vi "Relay_CYL.vi"(6 "DUT":u8, 7 "EOL/FCT":bool, 8 "error out":errorcluster, 9 "DOs":bool[](array[boolean]), 10 "Relay_Channel_Out":T1[](array[typedef]), 11 "Relay":refnum<queue>) -> (0 "error out 2":errorcluster)   [LabVIEW 2024, in "Test_2.lvlib"]
uses:
  Test_2.lvlib
  Relay_Module/support/Relay_Enum_OUT.ctl
  Relay_Module/Relay_Module.lvlib
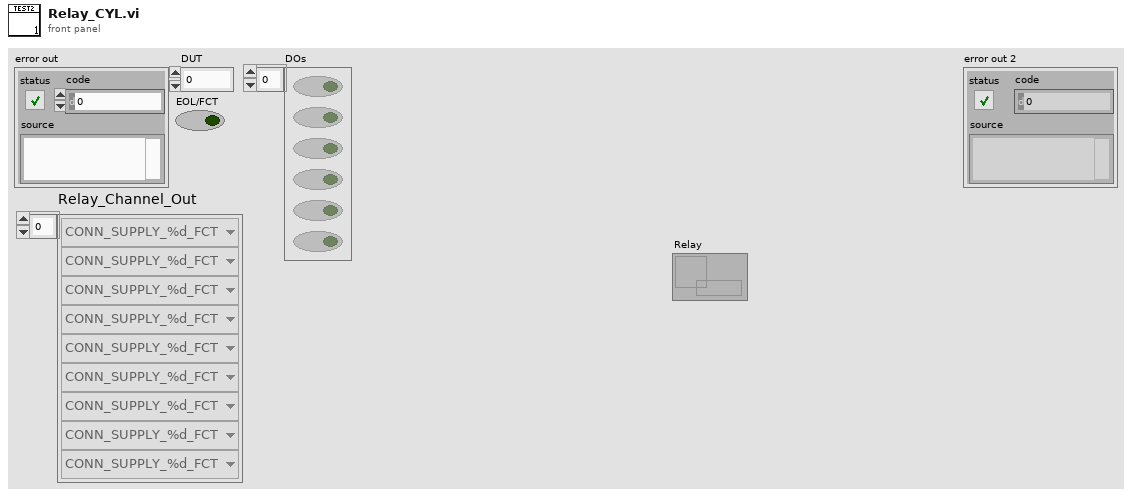
[diagram p1: front panel]
types:
  T1 = typedef "Relay_Module.lvlib/Relay_Enum_OUT.ctl" = enum16{"CONN_SUPPLY_%d_FCT", "HB_CONN_%d_FCT", "L_IND_CONN_%d_FCT", "R_IND_CONN_%d_FCT", "SW1_%d_FCT", "SW2_%d_FCT", "CAN_H_%d_FCT", "CAN_L_%d_FCT", "CYLINDER_ON/OFF_%d_FCT", "SPARE_1_%d_FCT", "SPARE_2_%d_FCT", "Tower Red", "Tower Amber", "Tower Green", "Tower Buzzer", "SLIMRELAY_DUT_%d_FCT", "GND_DMM_%d_EOL", "CAN_H_RES_%d_EOL", "CAN_L_RES_%d_EOL", "L_IND_RES_%d_EOL", "R_IND_RES_%d_EOL", "HB_CONN_DMM_%d_EOL", "14V_RES_%d_EOL", "CAN_L_(DMM-)_%d_EOL", "CAN_H_%d_EOL", "CAN_L_%d_EOL", "14V_%d_EOL", "GND_%d_EOL", "HB_CONN_%d_EOL", "L_IND_%d_EOL", "R_IND_%d_EOL", "CYLINDER_DUT_%d_EOL", "CYL_PB_1_%d_EOL", "CYL_PB_2_%d_EOL", "DUT_PASS_%d_EOL", "DUT_FAIL_%d_EOL", "SPARE1_%d_EOL", "Tower Red_EOL", "Tower Amber_EOL", "Tower Green_EOL", "Tower Buzzer_EOL"}
  T2 = cluster{"Message":string, "Message Data":variant}
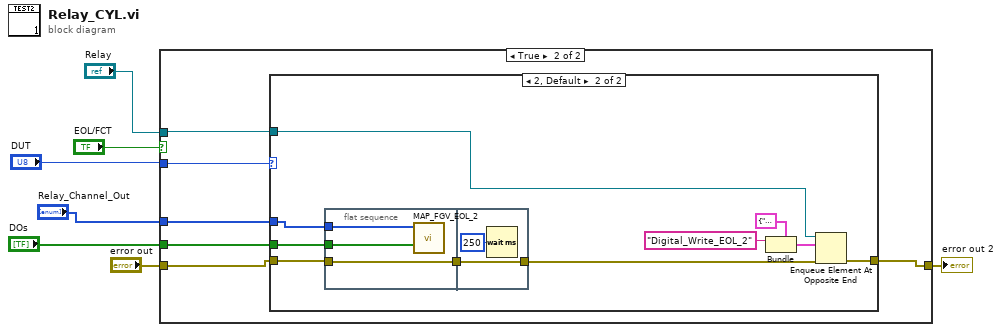
[diagram p0: block diagram]
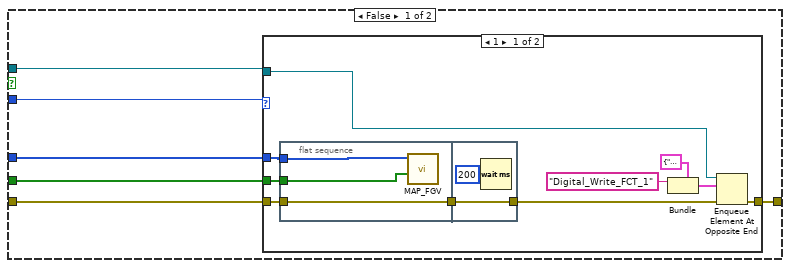
[diagram p2: hidden frame]
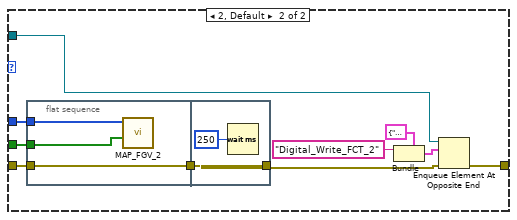
[diagram p3: hidden frame]
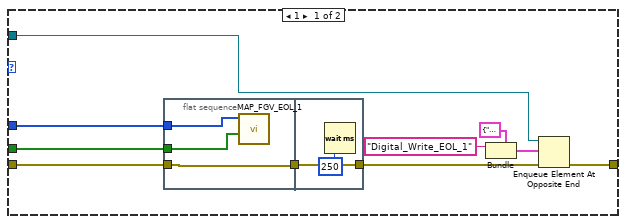
[diagram p4: hidden frame]
diagram:
  n1 = case shown="True" "EOL/FCT" {
    tunnel: "error out" -> [w13 w49]
    tunnel: [w12 w48] -> w1
    tunnel: "DUT" -> [w11 w47]
    tunnel: "Relay" -> [w10 w46]
    tunnel: "Relay_Channel_Out" -> [w9 w45]
    tunnel: "DOs" -> [w8 w44]
    frame False {
      n2 = case shown="1" w11 {
        tunnel: w13 -> [w19 w34]
        tunnel: [w23 w38] -> w12
        tunnel: w10 -> [w16 w31]
        tunnel: w9 -> [w15 w30]
        tunnel: w8 -> [w14 w29]
        frame 1 {
          n3 = flat-sequence {
            tunnel: w19 -> [w26]
            tunnel: [w26] -> w17
            tunnel: w15 -> [w25]
            tunnel: w14 -> [w24]
            tunnel: [w28] -> w18
            tunnel: w17 -> [w28]
            frame #0 {
              n4 = call "MAP_FGV.vi"("DOs"=w24, "Relay_Channel_Out"=w25) -> ()  [unwired: 7 in, 3 out]
            }
            frame #1 {
              n5 = Wait (ms)(milliseconds to wait=u32 200) -> ()  [unwired: 1 out]
            }
          }
          n6 = Bundle(cluster=T2 {"Message"="", "Message Data"=variant} ("element"), "Message"="Digital_Write_FCT_1") -> (w21:T2)  [unwired: 1 in]
          n7 = Enqueue Element At Opposite End(queue=w16, element=w21, error in (no error)=w18) -> (error out=w23:errorcluster)  [unwired: 1 in, 2 out]
        }
        frame 2, Default {
          n8 = flat-sequence {
            tunnel: w34 -> [w41]
            tunnel: [w41] -> w32
            tunnel: w30 -> [w40]
            tunnel: w29 -> [w39]
            tunnel: [w43] -> w33
            tunnel: w32 -> [w43]
            frame #0 {
              n9 = call "MAP_FGV_2.vi"("DOs"=w39, "Relay_Channel_Out"=w40) -> ()  [unwired: 7 in, 3 out]
            }
            frame #1 {
              n10 = Wait (ms)(milliseconds to wait=u32 250) -> ()  [unwired: 1 out]
            }
          }
          n11 = Bundle(cluster=T2 {"Message"="", "Message Data"=variant} ("element"), "Message"="Digital_Write_FCT_2") -> (w37:T2)  [unwired: 1 in]
          n12 = Enqueue Element At Opposite End(queue=w31, element=w37, error in (no error)=w33) -> (error out=w38:errorcluster)  [unwired: 1 in, 2 out]
        }
      }
    }
    frame True {
      n13 = case shown="2, Default" w47 {
        tunnel: w49 -> [w55 w70]
        tunnel: [w59 w74] -> w48
        tunnel: w46 -> [w52 w67]
        tunnel: w45 -> [w51 w66]
        tunnel: w44 -> [w50 w65]
        frame 1 {
          n14 = flat-sequence {
            tunnel: w55 -> [w62]
            tunnel: [w62] -> w53
            tunnel: w51 -> [w61]
            tunnel: w50 -> [w60]
            tunnel: [w64] -> w54
            tunnel: w53 -> [w64]
            frame #0 {
              n15 = call "MAP_FGV_EOL_1.vi"("DOs"=w60, "Relay_Channel_Out"=w61) -> ()  [unwired: 7 in, 3 out]
            }
            frame #1 {
              n16 = Wait (ms)(milliseconds to wait=u32 250) -> ()  [unwired: 1 out]
            }
          }
          n17 = Bundle(cluster=T2 {"Message"="", "Message Data"=variant} ("element"), "Message"="Digital_Write_EOL_1") -> (w58:T2)  [unwired: 1 in]
          n18 = Enqueue Element At Opposite End(queue=w52, element=w58, error in (no error)=w54) -> (error out=w59:errorcluster)  [unwired: 1 in, 2 out]
        }
        frame 2, Default {
          n19 = flat-sequence {
            tunnel: w70 -> [w77]
            tunnel: [w77] -> w68
            tunnel: w66 -> [w76]
            tunnel: w65 -> [w75]
            tunnel: [w79] -> w69
            tunnel: w68 -> [w79]
            frame #0 {
              n20 = call "MAP_FGV_EOL_2.vi"("DOs"=w75, "Relay_Channel_Out"=w76) -> ()  [unwired: 7 in, 3 out]
            }
            frame #1 {
              n21 = Wait (ms)(milliseconds to wait=u32 250) -> ()  [unwired: 1 out]
            }
          }
          n22 = Bundle(cluster=T2 {"Message"="", "Message Data"=variant} ("element"), "Message"="Digital_Write_EOL_2") -> (w73:T2)  [unwired: 1 in]
          n23 = Enqueue Element At Opposite End(queue=w67, element=w73, error in (no error)=w69) -> (error out=w74:errorcluster)  [unwired: 1 in, 2 out]
        }
      }
    }
  }
  "error out 2" <- w1
